vi "Get Event Reference.vi"(4 "error in (no error)":errorcluster) -> (0 "error out":errorcluster, 3 "Change Source":refnum<user-event>)   [LabVIEW 2015, in "Change Source.lvlib"]
uses:
  Change Source.lvlib
  _typedefs/Event Data.ctl
  _libraries/Startup Processes/_typedefs/Subpanel Names.ctl
  _libraries/Startup Processes/Startup Processes.lvlib
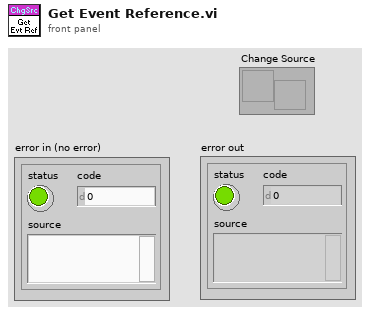
[diagram p1: front panel]
types:
  T1 = typedef "Change Source.lvlib/Event Data.ctl" = cluster{"Source Name":T2, "Save Button":refnum<vi>, "GUI Refnum":refnum<vi>, "Menu Refnum":refnum<k9>}
  T2 = typedef "Startup Processes.lvlib/Subpanel Names.ctl" = enum16{"Sine Source", "Ramp Source", "Hen House TC", "Dog House TC", "Out House TC"}
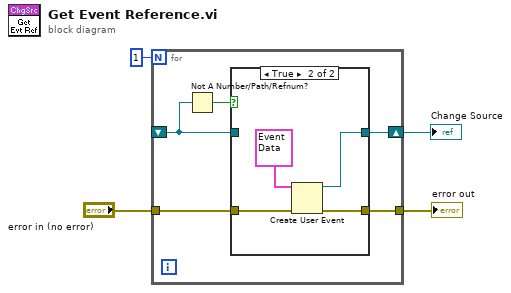
[diagram p0: block diagram]
diagram:
  n1 = for {
    N: 1 -> [_]
    shift-right: [w6] -> w4
    shift-left: _ -> [w8]
    tunnel: "error in (no error)" -> [w7]
    tunnel: [w5] -> w1
    n2 = Not A Number/Path/Refnum?(number/path/refnum=w8) -> (NaN/Path/Refnum?=w9:bool)
    n3 = case shown="True" w9 {
      tunnel: w8 -> [w11 _]
      tunnel: w7 -> [w10 w15]
      tunnel: [w11 w14] -> w6
      tunnel: [w10 w13] -> w5
      frame False {
      }
      frame True {
        n4 = Create User Event(user event datatype=T1 {"Source Name"=enum."Sine Source", "Save Button"=refnum, "GUI Refnum"=refnum, "Menu Refnum"=refnum} ("data"), error in=w15) -> (user event=w14:refnum<user-event>, error out=w13:errorcluster)
      }
    }
  }
  "error out" <- w1
  "Change Source" <- w4
